vi "create_custom_template.vi"() -> ()   [LabVIEW 2022 SP3]
uses:
  <vilib>/Utility/file.llb/Read Delimited Spreadsheet (string).vi
  <vilib>/Utility/file.llb/Write Delimited Spreadsheet (string).vi
panel:
  out "Table Control":string[][](table)=[["U/Uref", "W/Uref", "u^2/Uref^2", "w^2/Uref^2", "U", "W", "u^2", "w^2", "U/Uref", "W/Uref", "u^2/Uref^2", "w^2/Uref^2", "U", "W", "u^2", "w^2", "uw/Uref^2", "uw", "uw/Uref^2", "uw", "CUrefH^2/Q", "c^2(Uref/Q)^2", "", "c^2", "CUrefH^2/Q", "c^2(Uref/Q)^2", "", "c^2"], ["", "", "", "", "", "", "", "", "", "", "", "", "(m/s)", "(m/s)", "(m/s)^2", "(m/s)^2", "", "", "", "(m/s)^2", "", "", "", "", "", "", "", "(ppm)^2"], ["", "", "", "", "(m/s)", "(m/s)", "(m/s)^2", "(m/s)^2", "Std Error", "Std Error", "Std Error", "Std Error", "Std Error", "Std Error", "Std Error", "Std Error", "", "(m/s)^2", "Std Error", "Std Error", "", "", "", "(ppm)^2", "Std Error", "Std Error", "", "Std Error"], ["", "", "", "", "", "", "", "", "", "", "", "", "", "", "", "", "", "", "", "", "", "", "", "", "", "", "", ""], ["U/Uref::", "W/Uref::", "u^2/Uref^2::", "w^2/Uref^2::", "U::(m/s)", "W::(m/s)", "u^2::(m/s)^2", "w^2::(m/s)^2", "U/Uref::Std Error", "W/Uref::Std Error", "u^2/Uref^2::Std Error", "w^2/Uref^2::Std Error", "U:(m/s):Std Error", "W:(m/s):Std Error", "u^2:(m/s)^2:Std Error", "w^2:(m/s)^2:Std Error", "uw/Uref^2::", "uw::(m/s)^2", "uw/Uref^2::Std Error", "uw:(m/s)^2:Std Error", "CUrefH^2/Q::", "c^2(Uref/Q)^2::", "", "c^2::(ppm)^2", "CUrefH^2/Q::Std Error", "c^2(Uref/Q)^2::Std Error", "", "c^2:(ppm)^2:Std Error"], ["", "", "", "", "", "", "", "", "", "", "", "", "", "", "", "", "", "", "", "", "", "", "", "", "", "", "", ""], ["**Description Start**", "**Description Start**", "**Description Start**", "**Description Start**", "**Description Start**", "**Description Start**", "**Description Start**", "**Description Start**", "**Description Start**", "**Description Start**", "**Description Start**", "**Description Start**", "**Description Start**", "**Description Start**", "**Description Start**", "**Description Start**", "**Description Start**", "**Description Start**", "**Description Start**", "**Description Start**", "**Description Start**", "**Description Start**", "", "**Description Start**", "**Description Start**", "**Description Start**", "", "**Description Start**"], ["**Description End**", "**Description End**", "**Description End**", "**Description End**", "**Description End**", "**Description End**", "**Description End**", "**Description End**", "**Description End**", "**Description End**", "**Description End**", "**Description End**", "**Description End**", "**Description End**", "**Description End**", "**Description End**", "**Description End**", "**Description End**", "**Description End**", "**Description End**", "**Description End**", "**Description End**", "", "**Description End**", "**Description End**", "**Description End**", "", "**Description End**"], ["", "", "", "", "", "", "", "", "", "", "", "", "", "", "", "", "", "", "", "", "", "", "", "", "", "", "", ""], ["**Tolerance Start**", "**Tolerance Start**", "**Tolerance Start**", "**Tolerance Start**", "**Tolerance Start**", "**Tolerance Start**", "**Tolerance Start**", "**Tolerance Start**", "**Tolerance Start**", "**Tolerance Start**", "**Tolerance Start**", "**Tolerance Start**", "**Tolerance Start**", "**Tolerance Start**", "**Tolerance Start**", "**Tolerance Start**", "**Tolerance Start**", "**Tolerance Start**", "**Tolerance Start**", "**Tolerance Start**", "**Tolerance Start**", "**Tolerance Start**", "", "**Tolerance Start**", "**Tolerance Start**", "**Tolerance Start**", "", "**Tolerance Start**"], ["0.1", "1", "1", "1", "1", "1", "1", "1", "1", "1", "1", "1", "1", "1", "1", "1", "1", "1", "1", "1", "1", "1", "", "1", "1", "1", "", "1"], ["**Tolerance End**", "**Tolerance End**", "**Tolerance End**", "**Tolerance End**", "**Tolerance End**", "**Tolerance End**", "**Tolerance End**", "**Tolerance End**", "**Tolerance End**", "**Tolerance End**", "**Tolerance End**", "**Tolerance End**", "**Tolerance End**", "**Tolerance End**", "**Tolerance End**", "**Tolerance End**", "**Tolerance End**", "**Tolerance End**", "**Tolerance End**", "**Tolerance End**", "**Tolerance End**", "**Tolerance End**", "", "**Tolerance End**", "**Tolerance End**", "**Tolerance End**", "", "**Tolerance End**"], ["", "", "", "", "", "", "", "", "", "", "", "", "", "", "", "", "", "", "", "", "", "", "", "", "", "", "", ""], ["**Precision Start**", "**Precision Start**", "**Precision Start**", "**Precision Start**", "**Precision Start**", "**Precision Start**", "**Precision Start**", "**Precision Start**", "**Precision Start**", "**Precision Start**", "**Precision Start**", "**Precision Start**", "**Precision Start**", "**Precision Start**", "**Precision Start**", "**Precision Start**", "**Precision Start**", "**Precision Start**", "**Precision Start**", "**Precision Start**", "**Precision Start**", "**Precision Start**", "", "**Precision Start**", "**Precision Start**", "**Precision Start**", "", "**Precision Start**"], ["3", " ", " ", " ", " ", " ", " ", " ", " ", " ", " ", " ", " ", " ", " ", " ", " ", " ", " ", " ", " ", " ", "", " ", " ", " ", "", " "], ["**Precision End**", "**Precision End**", "**Precision End**", "**Precision End**", "**Precision End**", "**Precision End**", "**Precision End**", "**Precision End**", "**Precision End**", "**Precision End**", "**Precision End**", "**Precision End**", "**Precision End**", "**Precision End**", "**Precision End**", "**Precision End**", "**Precision End**", "**Precision End**", "**Precision End**", "**Precision End**", "**Precision End**", "**Precision End**", "", "**Precision End**", "**Precision End**", "**Precision End**", "", "**Precision End**"], ["", "", "", "", "", "", "", "", "", "", "", "", "", "", "", "", "", "", "", "", "", "", "", "", "", "", "", ""], ["**Dispose Start**", "**Dispose Start**", "**Dispose Start**", "**Dispose Start**", "**Dispose Start**", "**Dispose Start**", "**Dispose Start**", "**Dispose Start**", "**Dispose Start**", "**Dispose Start**", "**Dispose Start**", "**Dispose Start**", "**Dispose Start**", "**Dispose Start**", "**Dispose Start**", "**Dispose Start**", "**Dispose Start**", "**Dispose Start**", "**Dispose Start**", "**Dispose Start**", "**Dispose Start**", "**Dispose Start**", "", "**Dispose Start**", "**Dispose Start**", "**Dispose Start**", "", "**Dispose Start**"], ["If Blank", "If Blank", "If Blank", "If Blank", "If Blank", "If Blank", "If Blank", "If Blank", "If Blank", "If Blank", "If Blank", "If Blank", "If Blank", "If Blank", "If Blank", "If Blank", "If Blank", "If Blank", "If Blank", "If Blank", "If Blank", "If Blank", "", "If Blank", "If Blank", "If Blank", "", "If Blank"], ["**Dispose End**", "**Dispose End**", "**Dispose End**", "**Dispose End**", "**Dispose End**", "**Dispose End**", "**Dispose End**", "**Dispose End**", "**Dispose End**", "**Dispose End**", "**Dispose End**", "**Dispose End**", "**Dispose End**", "**Dispose End**", "**Dispose End**", "**Dispose End**", "**Dispose End**", "**Dispose End**", "**Dispose End**", "**Dispose End**", "**Dispose End**", "**Dispose End**", "", "**Dispose End**", "**Dispose End**", "**Dispose End**", "", "**Dispose End**"], ["", "", "", "", "", "", "", "", "", "", "", "", "", "", "", "", "", "", "", "", "", "", "", "", "", "", "", ""], ["**Summarise Start**", "**Summarise Start**", "**Summarise Start**", "**Summarise Start**", "**Summarise Start**", "**Summarise Start**", "**Summarise Start**", "**Summarise Start**", "**Summarise Start**", "**Summarise Start**", "**Summarise Start**", "**Summarise Start**", "**Summarise Start**", "**Summarise Start**", "**Summarise Start**", "**Summarise Start**", "**Summarise Start**", "**Summarise Start**", "**Summarise Start**", "**Summarise Start**", "**Summarise Start**", "**Summarise Start**", "", "**Summarise Start**", "**Summarise Start**", "**Summarise Start**", "", "**Summarise Start**"], ["FALSE", "FALSE", "FALSE", "FALSE", "FALSE", "FALSE", "FALSE", "FALSE", "FALSE", "FALSE", "FALSE", "FALSE", "FALSE", "FALSE", "FALSE", "FALSE", "FALSE", "FALSE", "FALSE", "FALSE", "FALSE", "FALSE", "", "FALSE", "FALSE", "FALSE", "", "FALSE"], ["**Summarise End**", "**Summarise End**", "**Summarise End**", "**Summarise End**", "**Summarise End**", "**Summarise End**", "**Summarise End**", "**Summarise End**", "**Summarise End**", "**Summarise End**", "**Summarise End**", "**Summarise End**", "**Summarise End**", "**Summarise End**", "**Summarise End**", "**Summarise End**", "**Summarise End**", "**Summarise End**", "**Summarise End**", "**Summarise End**", "**Summarise End**", "**Summarise End**", "", "**Summarise End**", "**Summarise End**", "**Summarise End**", "", "**Summarise End**"], ["", "", "", "", "", "", "", "", "", "", "", "", "", "", "", "", "", "", "", "", "", "", "", "", "", "", "", ""], ["**Source Start**", "**Source Start**", "**Source Start**", "**Source Start**", "**Source Start**", "**Source Start**", "**Source Start**", "**Source Start**", "**Source Start**", "**Source Start**", "**Source Start**", "**Source Start**", "**Source Start**", "**Source Start**", "**Source Start**", "**Source Start**", "**Source Start**", "**Source Start**", "**Source Start**", "**Source Start**", "**Source Start**", "**Source Start**", "", "**Source Start**", "**Source Start**", "**Source Start**", "", "**Source Start**"], ["U/Uref", "W/Uref", "u^2/U_{ref}^2", "w^2/U_{ref}^2::", "LDA (U):Mean:U", "LDA (W):Mean:W", "LDA (U):Variance:u^2", "LDA (W):Variance:w^2", "U/U(ref)::St Error", "W/U(ref)::St Error", "u^2/U_{ref}^2::St Error", "w^2/U_{ref}^2::St Error", "LDA (U):Mean U:Standard Error", "LDA (W):Standard Error:in Mean", "LDA (U):Standard Error:in Variance", "LDA (W):Standard Error:in Variance", "uw/U_{ref}^2::", "LDA (U) & LDA (W):Correlation:uw", "-uw/U_{ref}^2::St Error", "LDA (U) & LDA (W):Correlation uw:Standard Error", "CU/Q", "c'/C", "", "Ch 1:Variance:FF (C)", "CU/Q::Err", "c'U(ref)/Q:(m^{-2}):St Error", "", "FF (C):Standard Error:in Variance"], [" ", " ", " ", " ", "Do not prompt me if this channnel is not found", "Do not prompt me if this channnel is not found", "Do not prompt me if this channnel is not found", "Do not prompt me if this channnel is not found", " ", " ", " ", " ", "Do not prompt me if this channnel is not found", "LDA (W):Mean W:Standard Error", "LDA (U):Variance u^2:Standard Error", "LDA (W):Variance w^2:Standard Error", " ", "Do not prompt me if this channnel is not found", " ", "Do not prompt me if this channnel is not found", " ", " ", "", "FF (C):Variance:c^2", " ", " ", "", "FF (C):Variance c^2:Standard Error"], [" ", " ", " ", " ", " ", " ", " ", " ", " ", " ", " ", " ", " ", "Do not prompt me if this channnel is not found", "Do not prompt me if this channnel is not found", "Do not prompt me if this channnel is not found", " ", " ", " ", " ", " ", " ", "", "Do not prompt me if this channnel is not found", " ", " ", "", "Do not prompt me if this channnel is not found"], [" ", " ", " ", " ", " ", " ", " ", " ", " ", " ", " ", " ", " ", " ", " ", " ", " ", " ", " ", " ", " ", " ", "", " ", " ", " ", "", " "], ["**Source End**", "**Source End**", "**Source End**", "**Source End**", "**Source End**", "**Source End**", "**Source End**", "**Source End**", "**Source End**", "**Source End**", "**Source End**", "**Source End**", "**Source End**", "**Source End**", "**Source End**", "**Source End**", "**Source End**", "**Source End**", "**Source End**", "**Source End**", "**Source End**", "**Source End**", "", "**Source End**", "**Source End**", "**Source End**", "", "**Source End**"], ["", "", "", "", "", "", "", "", "", "", "", "", "", "", "", "", "", "", "", "", "", "", "", "", "", "", "", ""], ["**Replace Start**", "**Replace Start**", "**Replace Start**", "**Replace Start**", "**Replace Start**", "**Replace Start**", "**Replace Start**", "**Replace Start**", "**Replace Start**", "**Replace Start**", "**Replace Start**", "**Replace Start**", "**Replace Start**", "**Replace Start**", "**Replace Start**", "**Replace Start**", "**Replace Start**", "**Replace Start**", "**Replace Start**", "**Replace Start**", "**Replace Start**", "**Replace Start**", "", "**Replace Start**", "**Replace Start**", "**Replace Start**", "", "**Replace Start**"], [" ", " ", " ", " ", " ", " ", " ", " ", " ", " ", " ", " ", " ", " ", " ", " ", " ", " ", " ", " ", " ", " ", "", " ", " ", " ", "", " "], [" ", " ", " ", " ", " ", " ", " ", " ", " ", " ", " ", " ", " ", " ", " ", " ", " ", " ", " ", " ", " ", " ", "", " ", " ", " ", "", " "], [" ", " ", " ", " ", " ", " ", " ", " ", " ", " ", " ", " ", " ", " ", " ", " ", " ", " ", " ", " ", " ", " ", "", " ", " ", " ", "", " "], [" ", " ", " ", " ", " ", " ", " ", " ", " ", " ", " ", " ", " ", " ", " ", " ", " ", " ", " ", " ", " ", " ", "", " ", " ", " ", "", " "], [" ", " ", " ", " ", " ", " ", " ", " ", " ", " ", " ", " ", " ", " ", " ", " ", " ", " ", " ", " ", " ", " ", "", " ", " ", " ", "", " "], [" ", " ", " ", " ", " ", " ", " ", " ", " ", " ", " ", " ", " ", " ", " ", " ", " ", " ", " ", " ", " ", " ", "", " ", " ", " ", "", " "], [" ", " ", " ", " ", " ", " ", " ", " ", " ", " ", " ", " ", " ", " ", " ", " ", " ", " ", " ", " ", " ", " ", "", " ", " ", " ", "", " "], [" ", " ", " ", " ", " ", " ", " ", " ", " ", " ", " ", " ", " ", " ", " ", " ", " ", " ", " ", " ", " ", " ", "", " ", " ", " ", "", " "], [" ", " ", " ", " ", " ", " ", " ", " ", " ", " ", " ", " ", " ", " ", " ", " ", " ", " ", " ", " ", " ", " ", "", " ", " ", " ", "", " "], [" ", " ", " ", " ", " ", " ", " ", " ", " ", " ", " ", " ", " ", " ", " ", " ", " ", " ", " ", " ", " ", " ", "", " ", " ", " ", "", " "], [" ", " ", " ", " ", " ", " ", " ", " ", " ", " ", " ", " ", " ", " ", " ", " ", " ", " ", " ", " ", " ", " ", "", " ", " ", " ", "", " "], ["**Replace End**", "**Replace End**", "**Replace End**", "**Replace End**", "**Replace End**", "**Replace End**", "**Replace End**", "**Replace End**", "**Replace End**", "**Replace End**", "**Replace End**", "**Replace End**", "**Replace End**", "**Replace End**", "**Replace End**", "**Replace End**", "**Replace End**", "**Replace End**", "**Replace End**", "**Replace End**", "**Replace End**", "**Replace End**", "", "**Replace End**", "**Replace End**", "**Replace End**", "", "**Replace End**"], ["", "", "", "", "", "", "", "", "", "", "", "", "", "", "", "", "", "", "", "", "", "", "", "", "", "", "", ""], ["**Maths Start**", "**Maths Start**", "**Maths Start**", "**Maths Start**", "**Maths Start**", "**Maths Start**", "**Maths Start**", "**Maths Start**", "**Maths Start**", "**Maths Start**", "**Maths Start**", "**Maths Start**", "**Maths Start**", "**Maths Start**", "**Maths Start**", "**Maths Start**", "**Maths Start**", "**Maths Start**", "**Maths Start**", "**Maths Start**", "**Maths Start**", "**Maths Start**", "", "**Maths Start**", "**Maths Start**", "**Maths Start**", "", "**Maths Start**"], ["<<U::(m/s)>>/<<Uref::(m/s)>>", "<<W::(m/s)>>/<<Uref::(m/s)>>", "<<u^2::(m/s)^2>>/<<Uref::(m/s)>>^2", "<<w^2::(m/s)^2>>/<<Uref::(m/s)>>^2", " ", " ", " ", " ", "<<U:(m/s):Std Error>>/<<Uref::(m/s)>>", "<<W:(m/s):Std Error>>/<<Uref::(m/s)>>", "<<u^2:(m/s)^2:Std Error>>/<<Uref::(m/s)>>^2", "<<w^2:(m/s)^2:Std Error>>/<<Uref::(m/s)>>^2", " ", " ", " ", " ", "<<uw::(m/s)^2>>/<<Uref::(m/s)>>^2", " ", "<<uw:(m/s)^2:Std Error>>/<<Uref::(m/s)>>^2", " ", "<<C::(ppm)>>*<<UH^2/Q::>>", "<<c^2::(ppm)^2>>*<<UH^2/Q::>>^2", "", " ", "<<C:(ppm):Std Error>>*<<UH^2/Q::>>", "<<c^2:(ppm)^2:Std Error>>*<<UH^2/Q::>>^2", "", " "], [" ", " ", " ", " ", " ", " ", " ", " ", " ", " ", " ", " ", " ", " ", " ", " ", " ", " ", " ", " ", " ", " ", "", " ", " ", " ", "", " "], ["**Maths End**", "**Maths End**", "**Maths End**", "**Maths End**", "**Maths End**", "**Maths End**", "**Maths End**", "**Maths End**", "**Maths End**", "**Maths End**", "**Maths End**", "**Maths End**", "**Maths End**", "**Maths End**", "**Maths End**", "**Maths End**", "**Maths End**", "**Maths End**", "**Maths End**", "**Maths End**", "**Maths End**", "**Maths End**", "", "**Maths End**", "**Maths End**", "**Maths End**", "", "**Maths End**"], ["", "", "", "", "", "", "", "", "", "", "", "", "", "", "", "", "", "", "", "", "", "", "", "", "", "", "", ""], ["**Omit Start**", "**Omit Start**", "**Omit Start**", "**Omit Start**", "**Omit Start**", "**Omit Start**", "**Omit Start**", "**Omit Start**", "**Omit Start**", "**Omit Start**", "**Omit Start**", "**Omit Start**", "**Omit Start**", "**Omit Start**", "**Omit Start**", "**Omit Start**", "**Omit Start**", "**Omit Start**", "**Omit Start**", "**Omit Start**", "**Omit Start**", "**Omit Start**", "", "**Omit Start**", "**Omit Start**", "**Omit Start**", "", "**Omit Start**"], [" ", " ", " ", " ", " ", " ", " ", " ", " ", " ", " ", " ", " ", " ", " ", " ", " ", " ", " ", " ", " ", " ", "", " ", " ", " ", "", " "], [" ", " ", " ", " ", " ", " ", " ", " ", " ", " ", " ", " ", " ", " ", " ", " ", " ", " ", " ", " ", " ", " ", "", " ", " ", " ", "", " "], [" ", " ", " ", " ", " ", " ", " ", " ", " ", " ", " ", " ", " ", " ", " ", " ", " ", " ", " ", " ", " ", " ", "", " ", " ", " ", "", " "], ["**Omit End**", "**Omit End**", "**Omit End**", "**Omit End**", "**Omit End**", "**Omit End**", "**Omit End**", "**Omit End**", "**Omit End**", "**Omit End**", "**Omit End**", "**Omit End**", "**Omit End**", "**Omit End**", "**Omit End**", "**Omit End**", "**Omit End**", "**Omit End**", "**Omit End**", "**Omit End**", "**Omit End**", "**Omit End**", "", "**Omit End**", "**Omit End**", "**Omit End**", "", "**Omit End**"], ["", "", "", "", "", "", "", "", "", "", "", "", "", "", "", "", "", "", "", "", "", "", "", "", "", "", "", ""], ["**Folder level Start**", "**Folder level Start**", "**Folder level Start**", "**Folder level Start**", "**Folder level Start**", "**Folder level Start**", "**Folder level Start**", "**Folder level Start**", "**Folder level Start**", "**Folder level Start**", "**Folder level Start**", "**Folder level Start**", "**Folder level Start**", "**Folder level Start**", "**Folder level Start**", "**Folder level Start**", "**Folder level Start**", "**Folder level Start**", "**Folder level Start**", "**Folder level Start**", "**Folder level Start**", "**Folder level Start**", "", "**Folder level Start**", "**Folder level Start**", "**Folder level Start**", "", "**Folder level Start**"], ["**Folder level End**", "**Folder level End**", "**Folder level End**", "**Folder level End**", "**Folder level End**", "**Folder level End**", "**Folder level End**", "**Folder level End**", "**Folder level End**", "**Folder level End**", "**Folder level End**", "**Folder level End**", "**Folder level End**", "**Folder level End**", "**Folder level End**", "**Folder level End**", "**Folder level End**", "**Folder level End**", "**Folder level End**", "**Folder level End**", "**Folder level End**", "**Folder level End**", "", "**Folder level End**", "**Folder level End**", "**Folder level End**", "", "**Folder level End**"], ["", "", "", "", "", "", "", "", "", "", "", "", "", "", "", "", "", "", "", "", "", "", "", "", "", "", "", ""], ["**Minimum Value Start**", "**Minimum Value Start**", "**Minimum Value Start**", "**Minimum Value Start**", "**Minimum Value Start**", "**Minimum Value Start**", "**Minimum Value Start**", "**Minimum Value Start**", "**Minimum Value Start**", "**Minimum Value Start**", "**Minimum Value Start**", "**Minimum Value Start**", "**Minimum Value Start**", "**Minimum Value Start**", "**Minimum Value Start**", "**Minimum Value Start**", "**Minimum Value Start**", "**Minimum Value Start**", "**Minimum Value Start**", "**Minimum Value Start**", "**Minimum Value Start**", "**Minimum Value Start**", "", "**Minimum Value Start**", "**Minimum Value Start**", "**Minimum Value Start**", "", "**Minimum Value Start**"], ["**Minimum Value End**", "**Minimum Value End**", "**Minimum Value End**", "**Minimum Value End**", "**Minimum Value End**", "**Minimum Value End**", "**Minimum Value End**", "**Minimum Value End**", "**Minimum Value End**", "**Minimum Value End**", "**Minimum Value End**", "**Minimum Value End**", "**Minimum Value End**", "**Minimum Value End**", "**Minimum Value End**", "**Minimum Value End**", "**Minimum Value End**", "**Minimum Value End**", "**Minimum Value End**", "**Minimum Value End**", "**Minimum Value End**", "**Minimum Value End**", "", "**Minimum Value End**", "**Minimum Value End**", "**Minimum Value End**", "", "**Minimum Value End**"], ["", "", "", "", "", "", "", "", "", "", "", "", "", "", "", "", "", "", "", "", "", "", "", "", "", "", "", ""], ["**Maximum Value Start**", "**Maximum Value Start**", "**Maximum Value Start**", "**Maximum Value Start**", "**Maximum Value Start**", "**Maximum Value Start**", "**Maximum Value Start**", "**Maximum Value Start**", "**Maximum Value Start**", "**Maximum Value Start**", "**Maximum Value Start**", "**Maximum Value Start**", "**Maximum Value Start**", "**Maximum Value Start**", "**Maximum Value Start**", "**Maximum Value Start**", "**Maximum Value Start**", "**Maximum Value Start**", "**Maximum Value Start**", "**Maximum Value Start**", "**Maximum Value Start**", "**Maximum Value Start**", "", "**Maximum Value Start**", "**Maximum Value Start**", "**Maximum Value Start**", "", "**Maximum Value Start**"], ["**Maximum Value End**", "**Maximum Value End**", "**Maximum Value End**", "**Maximum Value End**", "**Maximum Value End**", "**Maximum Value End**", "**Maximum Value End**", "**Maximum Value End**", "**Maximum Value End**", "**Maximum Value End**", "**Maximum Value End**", "**Maximum Value End**", "**Maximum Value End**", "**Maximum Value End**", "**Maximum Value End**", "**Maximum Value End**", "**Maximum Value End**", "**Maximum Value End**", "**Maximum Value End**", "**Maximum Value End**", "**Maximum Value End**", "**Maximum Value End**", "", "**Maximum Value End**", "**Maximum Value End**", "**Maximum Value End**", "", "**Maximum Value End**"], ["", "", "", "", "", "", "", "", "", "", "", "", "", "", "", "", "", "", "", "", "", "", "", "", "", "", "", ""], ["**Ignore When Start**", "**Ignore When Start**", "**Ignore When Start**", "**Ignore When Start**", "**Ignore When Start**", "**Ignore When Start**", "**Ignore When Start**", "**Ignore When Start**", "**Ignore When Start**", "**Ignore When Start**", "**Ignore When Start**", "**Ignore When Start**", "**Ignore When Start**", "**Ignore When Start**", "**Ignore When Start**", "**Ignore When Start**", "**Ignore When Start**", "**Ignore When Start**", "**Ignore When Start**", "**Ignore When Start**", "**Ignore When Start**", "**Ignore When Start**", "", "**Ignore When Start**", "**Ignore When Start**", "**Ignore When Start**", "", "**Ignore When Start**"], [" ", " ", " ", " ", " ", " ", " ", " ", " ", " ", " ", " ", " ", " ", " ", " ", " ", " ", " ", " ", " ", " ", "", " ", " ", " ", "", " "], ["**Ignore When End**", "**Ignore When End**", "**Ignore When End**", "**Ignore When End**", "**Ignore When End**", "**Ignore When End**", "**Ignore When End**", "**Ignore When End**", "**Ignore When End**", "**Ignore When End**", "**Ignore When End**", "**Ignore When End**", "**Ignore When End**", "**Ignore When End**", "**Ignore When End**", "**Ignore When End**", "**Ignore When End**", "**Ignore When End**", "**Ignore When End**", "**Ignore When End**", "**Ignore When End**", "**Ignore When End**", "", "**Ignore When End**", "**Ignore When End**", "**Ignore When End**", "", "**Ignore When End**"]]
  out "Array 2":string[](array[string])=["U/Uref::", "W/Uref::", "u^2/Uref^2::", "w^2/Uref^2::", "U::(m/s)", "W::(m/s)", "u^2::(m/s)^2", "w^2::(m/s)^2", "U/Uref::Std Error", "W/Uref::Std Error", "u^2/Uref^2::Std Error", "w^2/Uref^2::Std Error", "U:(m/s):Std Error", "W:(m/s):Std Error", "u^2:(m/s)^2:Std Error", "w^2:(m/s)^2:Std Error", "uw/Uref^2::", "uw::(m/s)^2", "uw/Uref^2::Std Error", "uw:(m/s)^2:Std Error", "CUrefH^2/Q::", "c^2(Uref/Q)^2::", "C::(ppm)^2", "c^2::(ppm)^2", "CUrefH^2/Q::Std Error", "c^2(Uref/Q)^2::Std Error", "C:(ppm)^2:Std Error", "c^2:(ppm)^2:Std Error"]
  in  "Pressure":enum16{"None", "Uncorrelated", "Correlated"}(ring)
  in  "Velocity components":string="UW"
  in  "Concentration":enum16{"None", "Uncorrelated", "Correlated"}(ring)=enum."Uncorrelated"
  in  "File to create":path=path "C:/EnFlo Software/Data plotting/Creating Template files/Empty_Template.xls"
  in  "Full File":path=path "C:/EnFlo Software/Data plotting/Creating Template files/MAGIC_Full_Template.xls"
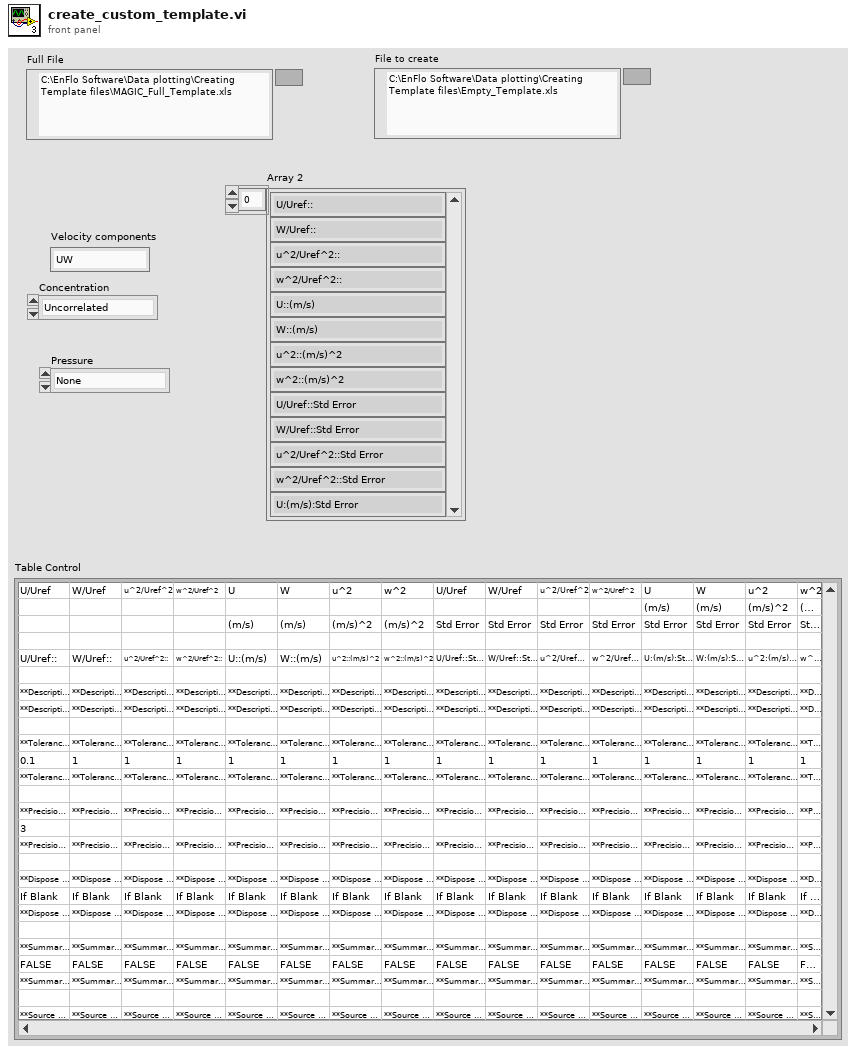
[diagram p1: front panel]
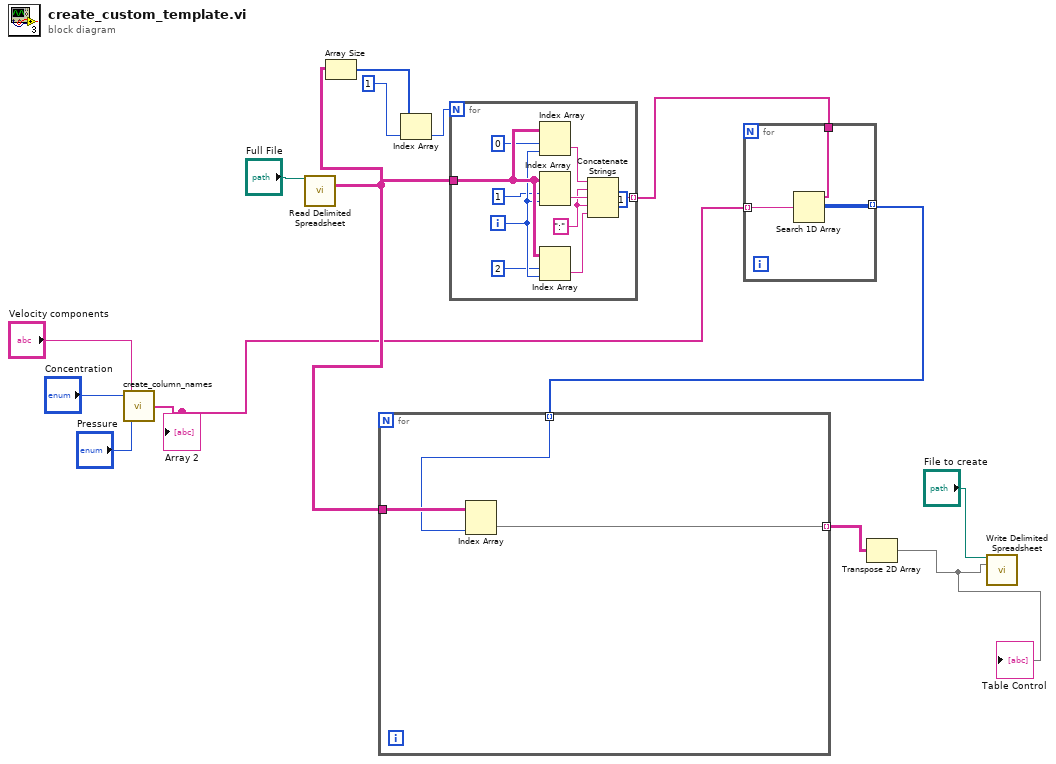
[diagram p0: block diagram]
diagram:
  (unwired) 11 ("index of element")
  n1 = call "create_column_names.vi"("Pressure"="Pressure", "Velocity components"="Velocity components", "Concentration"="Concentration") -> ("Array"=w5:string[])
  "Array 2" <- w5
  n2 = call-poly <vilib>:"Read Delimited Spreadsheet.vi"("file path (dialog if empty)"="Full File") -> ("all rows"=w6:string[][])  [unwired: 9 in, 5 out]
  n3 = Array Size(array=w6) -> (size(s)=w13:i32[])
  n4 = Index Array(array=w13, index=1) -> (element=w11:i32)
  n5 = for {
    N: w11 -> [_]
    tunnel: w6 -> [w24]
    tunnel: [w16] -> w10 mode=indexing
    i -> [w23]
    w15 = ":"
    n6 = Index Array(array=w24, index (row)=0 ("disabled index (row)"), index (col)=w23) -> (element=w19:string)
    n7 = Index Array(array=w24, index (row)=1 ("disabled index (row)"), index (col)=w23) -> (element=w18:string)
    n8 = Index Array(array=w24, index (row)=2 ("disabled index (row)"), index (col)=w23) -> (element=w17:string)
    n9 = Concatenate Strings(w19, w15, w18, w15, w17) -> (w16:string)
  }
  n10 = for {
    tunnel: w10 -> [w27]
    tunnel: w5 -> [w26] mode=indexing
    tunnel: [w25] -> w8 mode=indexing
    n11 = Search 1D Array(1D array=w27, element=w26) -> (index of element=w25:i32)  [unwired: 1 in]
  }
  n12 = for {
    tunnel: w8 -> [w29] mode=indexing
    tunnel: w6 -> [w30]
    tunnel: [w28] -> w7 mode=indexing
    n13 = Index Array(array=w30, index (col)=w29) -> (element=w28:string[])  [unwired: 1 in]
  }
  n14 = Transpose 2D Array(2D array=w7) -> (transposed array=w1:string[][])
  "Table Control" <- w1
  n15 = call-poly <vilib>:"Write Delimited Spreadsheet.vi"("file path (dialog if empty)"="File to create", "2D data"=w1) -> ()  [unwired: 12 in, 2 out]
